vi "I-O Test_010912025.vi"() -> ()   [LabVIEW 2021, in "Test VIs.lvclass"]
uses:
  Test VIs/Test VIs.lvclass
  Classes/Controller/I-O/I-O.lvclass
  Classes/Controller/Controller.lvclass
panel:
  out "Compression Sensor":bool=TRUE
  out "Sensor Channel":dbl
  out "Sensor":bool=TRUE
  out "sensor pin number":i32
  out "tray sensor":bool
  out "secondary valve sensor":bool
  out "primary valve sensor":bool
  in  "Turn on secondary vacuum":bool
  in  "turn on primary vacuum":bool
  in  "secure tray":bool
  out "Valve Channel":dbl
  in  "Type":enum16{"O ring Vac", "Baseplate Vac"}(ring)
  in  "Position":i32
  in  "Region":i32
  in  "On/Off":bool
  in  "Stop":bool
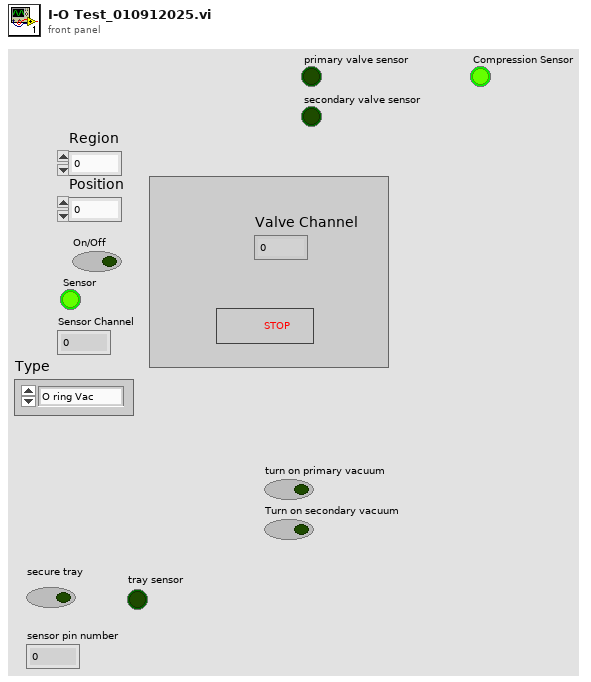
[diagram p1: front panel]
types:
  T1 = typedef "Controller.lvclass/Controllers.ctl" = cluster{"I-O.lvclass":refnum<class "I-O.lvclass">, "Gantry":refnum<k24>, "Dispenser":refnum<visa-resource-name>}
  T2 = typedef "I-O.lvclass/Pin Map.ctl" = cluster{"Region Valves":i32[], "Extra Valves":dbl[][][], "Tool Primary Valve":i32, "Tool Secondary Valve":i32, "Region Sensors":i32[], "Extra Sensors":dbl[][][], "Tool Primary Sensor":dbl, "Tool Secondary Sensor":dbl, "Compression Sensor":dbl, "5V":i32, "Dispenser Sensor":dbl, "Light Curtain":i32}
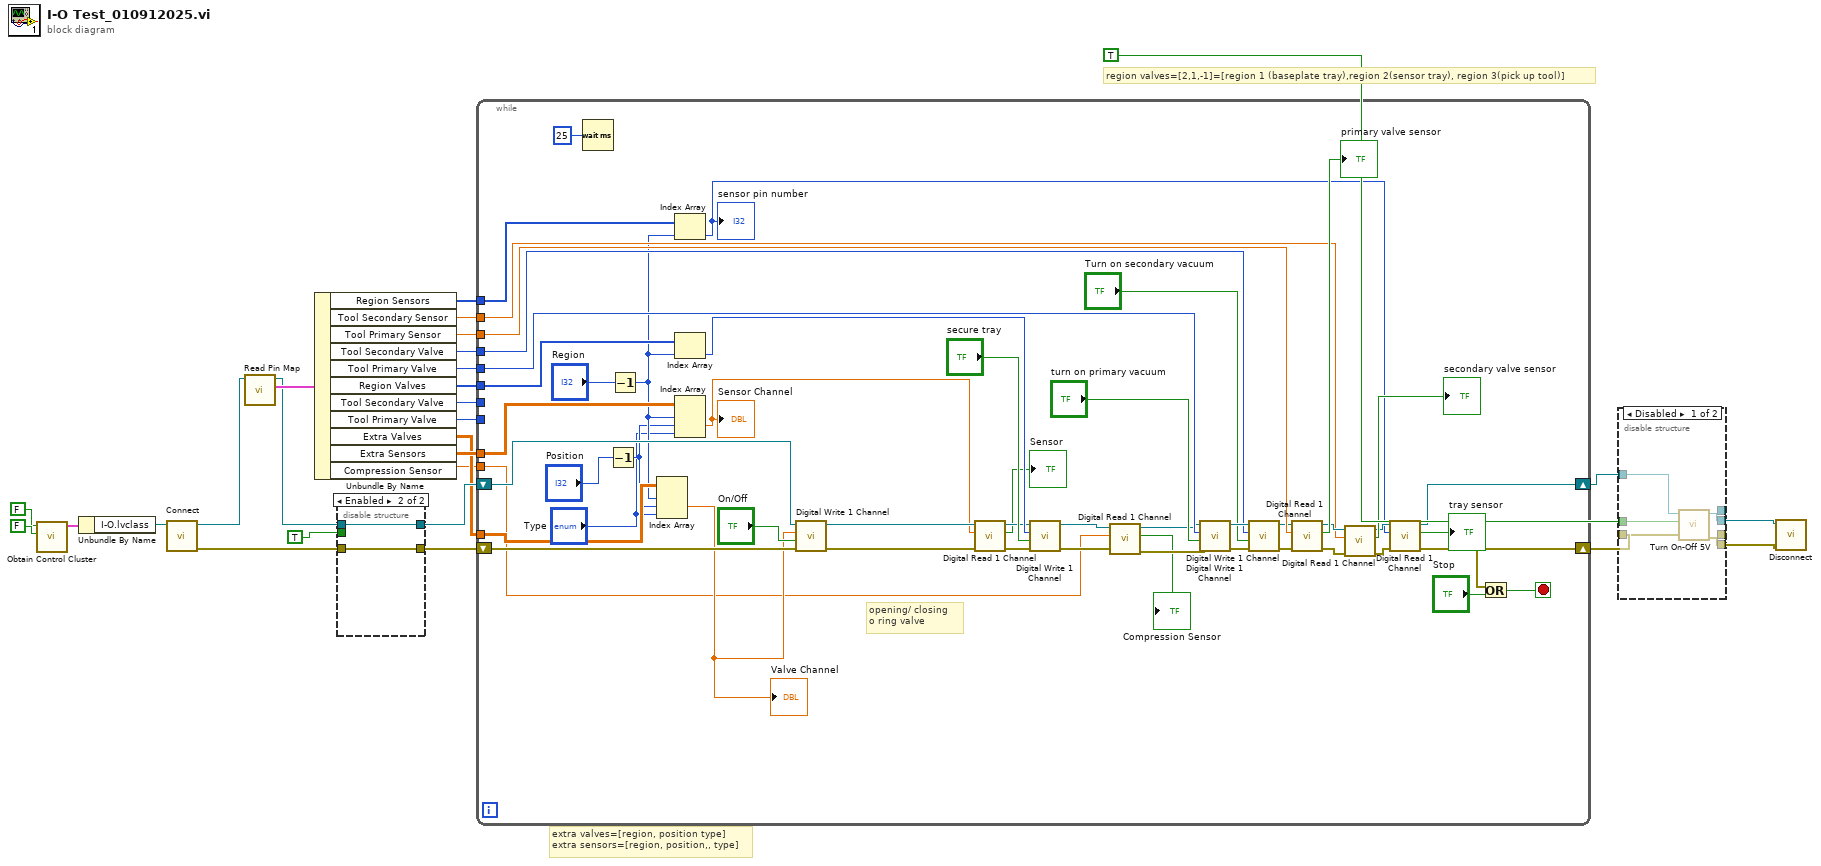
[diagram p0: block diagram]
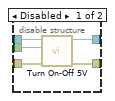
[diagram p2: hidden frame]
diagram:
  # "extra valves=[region, position type]\nextra sensors=[region, position,, type]"
  # "region valves=[2,1,-1]=[region 1 (baseplate tray),region 2(sensor tray), region 3(pick up tool)]"
  n1 = call "Obtain Control Cluster.vi"("Dispense"=FALSE, "Motion"=FALSE) -> ("Control Out"=w15:T1)  [unwired: 8 in, 1 out]
  n2 = Unbundle By Name(w15) -> ("I-O.lvclass"=w14:refnum<class "I-O.lvclass">)
  n3 = call-dynamic "Connect.vi"("Controller in"=w14) -> ("error out"=w20:errorcluster, "Controller out"=w22:refnum<class "I-O.lvclass">)  [unwired: 9 in]
  n4 = call-dynamic "Read Pin Map.vi"("I-O in"=w22) -> ("Pin Map 2"=w24:T2, "I-O out"=w23:refnum<class "I-O.lvclass">)  [unwired: 8 in, 1 out]
  n5 = Unbundle By Name(w24) -> ("Region Sensors"=w5:i32[], "Tool Secondary Sensor"=w6:dbl, "Tool Primary Sensor"=w7:dbl, "Tool Secondary Valve"=w8:i32, "Tool Primary Valve"=w9:i32, "Region Valves"=w10:i32[], "Tool Secondary Valve"=w12:i32, "Tool Primary Valve"=w11:i32, "Extra Valves"=w18:dbl[][][], "Extra Sensors"=w21:dbl[][][], "Compression Sensor"=w13:dbl)
  n6 = disable-structure shown="Enabled" {
    disable-tunnel: [w32 w34] -> w27
    disable-tunnel: TRUE ("Value") -> [w31 _]
    disable-tunnel: w23 -> [w30 w34]
    disable-tunnel: w20 -> [w29 w33]
    disable-tunnel: [w28 w33] -> w19
    frame Disabled {
      n7 = call-dynamic "Turn On-Off 5V.vi"("error in (no error)"=w29, "Value"=w31, "I-O in"=w30) -> ("error out"=w28:errorcluster, "I-O out"=w32:refnum<class "I-O.lvclass">)  [unwired: 7 in]
    }
    frame Enabled {
    }
  }
  n8 = while {
    shift-right: [w54] -> w25
    shift-left: w27 -> [w81]
    tunnel: w21 -> [w45]
    shift-right: [w56] -> w4
    shift-left: w19 -> [w80]
    tunnel: w18 -> [w46]
    tunnel: w13 -> [w36]
    tunnel: w12 -> [_]
    tunnel: w11 -> [_]
    tunnel: w10 -> [w75]
    tunnel: w9 -> [w72]
    tunnel: w8 -> [w69]
    tunnel: w7 -> [w66]
    tunnel: w6 -> [w61]
    tunnel: w5 -> [w58]
    stop <- w82 stop-if-true
    # "opening/ closing \no ring valve"
    n9 = Wait (ms)(milliseconds to wait=u32 25) -> ()  [unwired: 1 out]
    n10 = Decrement(x="Position") -> (x-1=w43:i32)
    n11 = Decrement(x="Region") -> (x-1=w44:i32)
    n12 = Index Array "Index Array"(array=w46, index (dim 0)=w44, index (dim 1)=w43, index (dim 2)="Type") -> (element=w76:dbl)
    "Valve Channel" <- w76
    n13 = Index Array(array=w58, index=w44) -> (element=w53:i32)
    "sensor pin number" <- w53
    n14 = Index Array(array=w75, index=w44) -> (element=w74:i32)
    n15 = Index Array(array=w45, index (dim 0)=w44, index (dim 1)=w43, index (dim 2)="Type") -> (element=w41:dbl)
    "Sensor Channel" <- w41
    n16 = call-dynamic "Digital Write 1 Channel.vi"("error constant"=w80, "Value"="On/Off", "Channel"=w76, "I-O.lvclass"=w81) -> ("error IO"=w50:errorcluster, "I-O.lvclass 2"=w51:refnum<class "I-O.lvclass">)  [unwired: 6 in]
    n17 = call-dynamic "Digital Read 1 Channel.vi"("error in (no error)"=w50, "Read"=w41, "I-O in"=w51) -> ("error out"=w49:errorcluster, "Value"=→"Sensor":bool, "I-O out"=w48:refnum<class "I-O.lvclass">)  [unwired: 6 in]
    n18 = call-dynamic "Digital Write 1 Channel.vi"("error constant"=w49, "Value"="secure tray", "Channel"=w74, "I-O.lvclass"=w48) -> ("error IO"=w40:errorcluster, "I-O.lvclass 2"=w39:refnum<class "I-O.lvclass">)  [unwired: 6 in]
    n19 = call-dynamic "Digital Read 1 Channel.vi"("error in (no error)"=w40, "Read"=w36, "I-O in"=w39) -> ("error out"=w37:errorcluster, "Value"=→"Compression Sensor":bool, "I-O out"=w38:refnum<class "I-O.lvclass">)  [unwired: 6 in]
    n20 = call-dynamic "Digital Write 1 Channel.vi"("error constant"=w37, "Value"="turn on primary vacuum", "Channel"=w72, "I-O.lvclass"=w38) -> ("error IO"=w67:errorcluster, "I-O.lvclass 2"=w70:refnum<class "I-O.lvclass">)  [unwired: 6 in]
    n21 = call-dynamic "Digital Write 1 Channel.vi"("error constant"=w67, "Value"="Turn on secondary vacuum", "Channel"=w69, "I-O.lvclass"=w70) -> ("error IO"=w63:errorcluster, "I-O.lvclass 2"=w65:refnum<class "I-O.lvclass">)  [unwired: 6 in]
    n22 = call-dynamic "Digital Read 1 Channel.vi"("error in (no error)"=w63, "Read"=w66, "I-O in"=w65) -> ("error out"=w59:errorcluster, "Value"=→"primary valve sensor":bool, "I-O out"=w62:refnum<class "I-O.lvclass">)  [unwired: 6 in]
    n23 = call-dynamic "Digital Read 1 Channel.vi"("error in (no error)"=w59, "Read"=w61, "I-O in"=w62) -> ("error out"=w57:errorcluster, "Value"=→"secondary valve sensor":bool, "I-O out"=w55:refnum<class "I-O.lvclass">)  [unwired: 6 in]
    n24 = call-dynamic "Digital Read 1 Channel.vi"("error in (no error)"=w57, "Read"=w53, "I-O in"=w55) -> ("error out"=w56:errorcluster, "Value"=→"tray sensor":bool, "I-O out"=w54:refnum<class "I-O.lvclass">)  [unwired: 6 in]
    n25 = Or(x=w56, y="Stop") -> (x .or. y?=w82:bool)
  }
  n26 = disable-structure shown="Disabled" {
    disable-tunnel: [_ w91] -> _
    disable-tunnel: w25 -> [w87 w91]
    disable-tunnel: [_ w90] -> _
    disable-tunnel: w4 -> [w89 w90]
    disable-tunnel: TRUE ("Value") -> [w88 _]
    disable-tunnel: [w86 _] -> w2
    disable-tunnel: [w85 _] -> w1
    frame Disabled {
      n27 = call-dynamic "Turn On-Off 5V.vi"("error in (no error)"=w89, "Value"=w88, "I-O in"=w87) -> ("error out"=w86:errorcluster, "I-O out"=w85:refnum<class "I-O.lvclass">)  [unwired: 7 in]
    }
    frame Enabled {
    }
  }
  n28 = call-dynamic "Disconnect.vi"("error in (no error)"=w2, "I-O in"=w1) -> ()  [unwired: 8 in, 1 out]
